vi "Base2_Init.vi"(8 "Error In":errorcluster, 11 "object in":refnum<class "Base2.lvclass">) -> (0 "Error Out":errorcluster, 3 "object out":refnum<class "Base2.lvclass">)   [LabVIEW 2020, in "Base2.lvclass"]
uses:
  Base2.lvclass
  Base2.lvclass/Base2.ctl
  Base1_class/Base1.lvclass
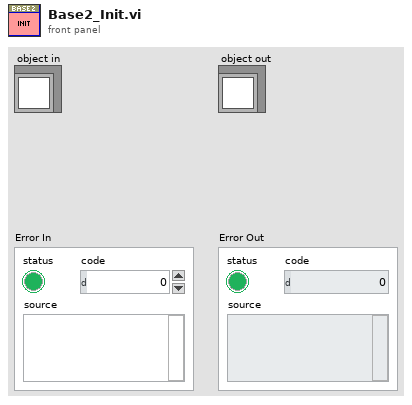
[diagram p1: front panel]
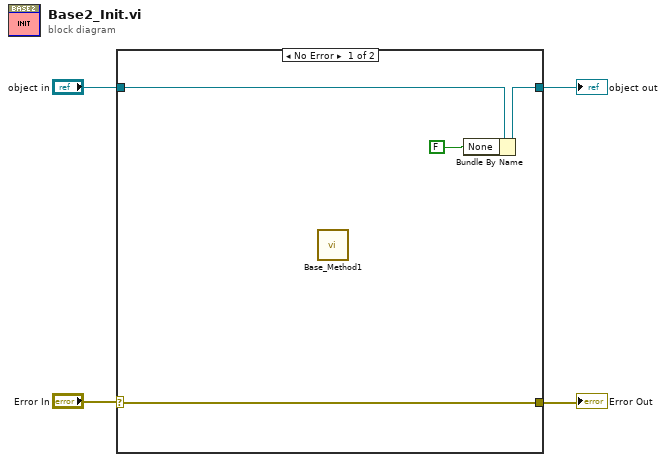
[diagram p0: block diagram]
diagram:
  n1 = case shown="No Error" "Error In" {
    selector: "Error In" -> [w5 w9]
    tunnel: "object in" -> [w8 w10]
    tunnel: [w7 w10] -> w3
    tunnel: [w5 w9] -> w1
    frame No Error {
      n2 = call "Base_Method1.vi"() -> ()  [unwired: 10 in, 2 out]
      n3 = Bundle By Name(cluster=w8, "None"=FALSE) -> (w7:refnum<class "Base2.lvclass">)
    }
    frame Error {
    }
  }
  "object out" <- w3
  "Error Out" <- w1
